vi "merFISH_init_ramp.vi"(2 "Total # z steps":i32, 3 "error in":errorcluster, 4 "Piezo queue":refnum<queue>, 5 "DAQ queue":refnum<queue>) -> (0 "error out":errorcluster, 1 "Piezo queue out":refnum<queue>)   [LabVIEW 2015]
uses:
  CONTROLS/Q_MCL_piezo_element.ctl
  CONTROLS/Q_DAQ_element.ctl
  GLOBAL/Global_DAQ.vi
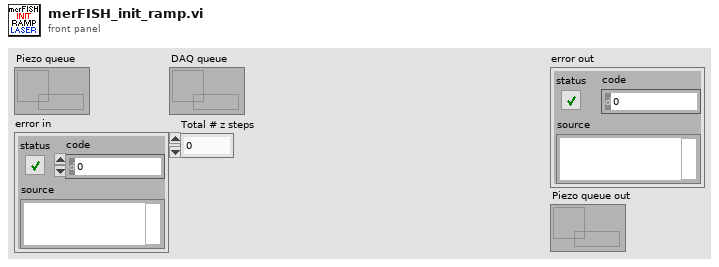
[diagram p1: front panel]
types:
  T1 = typedef "Q_DAQ_element.ctl" = cluster{"variant":variant, "Instruction":enum16{"DAQ_idle", "DAQ_initialize", "DAQ_error", "DAQ_security_stop", "DAQ_init_single_scan", "DAQ_single_scan", "DAQ_two_way_valve", "DAQ_init_merFISH", "DAQ_scan_merFISH", "DAQ_photobleaching_merFISH", "DAQ_close_merFISH", "DAQ_stop"}}
  T2 = typedef "Q_MCL_piezo_element.ctl" = cluster{"variant":variant, "Instruction":enum16{"Piezo_idle", "Piezo_initialize", "Piezo_error", "Piezo_security_stop", "Piezo_read_z", "Piezo_move_z", "Piezo_keyboard_move", "Piezo_close_autofocus_calibration_ramp", "Piezo_change_init_state", "Piezo_init_autofocus", "Piezo_init_autofocus_merFISH_TL", "Piezo_autofocus", "Piezo_autofocus_merFISH_TL", "Piezo_stop_autofocus", "Piezo_stop_autofocus_merFISH_TL", "Piezo_autofocus_lost", "Piezo_resume_autofocus_merFISH_TL", "Piezo_check_z_position_merFISH_TL", "Piezo_init_ramp", "Piezo_move_z_ramp", "Piezo_close_ramp", "Piezo_close_merFISH", "Piezo_stop"}}
  T3 = enum16{"DAQ_idle", "DAQ_initialize", "DAQ_error", "DAQ_security_stop", "DAQ_start_QPD", "DAQ_change_QPD_display", "DAQ_read_display_QPD_signal", "DAQ_QPD_init_autofocus", "DAQ_read_display_send_QPD_signal", "DAQ_close_autofocus_calibration_ramp", "DAQ_close_autofocus", "DAQ_405", "DAQ_488", "DAQ_561", "DAQ_641", "DAQ_zero_all", "DAQ_init_single_scan", "DAQ_single_scan", "DAQ_two_way_valve", "DAQ_init_merFISH", "DAQ_scan_merFISH", "DAQ_photobleaching_merFISH", "DAQ_close_merFISH", "DAQ_init_TL", "DAQ_synchro_TL", "DAQ_close_task_TL", "DAQ_close_TL", "DAQ_stop"}
  T4 = enum16{"DAQ_idle", "DAQ_initialize", "DAQ_error", "DAQ_security_stop", "DAQ_init_single_scan", "DAQ_single_scan", "DAQ_two_way_valve", "DAQ_init_merFISH", "DAQ_scan_merFISH", "DAQ_photobleaching_merFISH", "DAQ_close_merFISH", "DAQ_stop"}
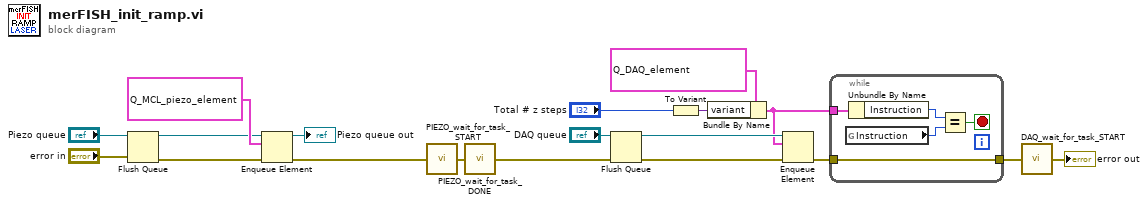
[diagram p0: block diagram]
diagram:
  n1 = Flush Queue(queue="Piezo queue", error in (no error)="error in") -> (queue out=w16:refnum<queue>, error out=w15:errorcluster)  [unwired: 1 out]
  n2 = Enqueue Element(queue=w16, element=T2 {"variant"=variant, "Instruction"=enum."Piezo_init_ramp"} ("Q_MCL_Piezo"), error in (no error)=w15) -> (queue out=→"Piezo queue out":refnum<queue>, error out=w19:errorcluster)  [unwired: 1 in, 1 out]
  n3 = call "PIEZO_wait_for_task_START.vi"("error in"=w19) -> ("error out"=w18:errorcluster)
  n4 = call "PIEZO_wait_for_task_DONE.vi"("error in"=w18) -> ("error out"=w12:errorcluster)
  n5 = Flush Queue(queue="DAQ queue", error in (no error)=w12) -> (queue out=w11:refnum<queue>, error out=w13:errorcluster)  [unwired: 1 out]
  n6 = To Variant(anything="Total # z steps") -> (Variant=w6:variant)
  n7 = Bundle By Name(cluster=T1 {"variant"=variant, "Instruction"=enum."DAQ_scan_merFISH"} ("Q_DAQ"), "variant"=w6) -> (w1:T1)
  n8 = Enqueue Element(queue=w11, element=w1, error in (no error)=w13) -> (error out=w3:errorcluster)  [unwired: 1 in, 2 out]
  n9 = while {
    tunnel: w3 -> [w21]
    tunnel: [w21] -> w2
    tunnel: w1 -> [w20]
    stop <- w23 stop-if-true
    n10 = global read "Global_DAQ.vi" "Instruction"() -> (w24:T3)
    n11 = Unbundle By Name(w20) -> ("Instruction"=w22:T4)
    n12 = Equal?(x=w22, y=w24) -> (x = y?=w23:bool)
  }
  n13 = call "DAQ_wait_for_task_START.vi"("error in"=w2) -> ("error out"=→"error out":errorcluster)
